vi "FRCts20_Backend_RemoveTeamEntry.vi"(8 "error in (no error)":errorcluster, 10 "Team Number":u16) -> (0 "error out":errorcluster, 2 "Status?":string)   [LabVIEW 2014, in "FRCts20_Backend_WebMethods.lvlib"]
doc: "RemoveTeam will eliminate a team from the superceding data set. All team information will be deleted."
uses:
  FRCts20_Backend_WebMethods.lvlib
  FRCts20_Backend_FGVOperation.ctl
  FRCts20_Backend_Engine.lvlib
panel:
  # "RemoveTeam will eliminate a team from the \nsuperceding data set. All team information\nwill be deleted."
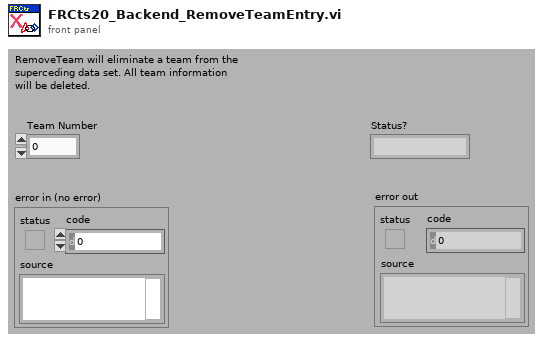
[diagram p1: front panel]
types:
  T1 = typedef "FRCts20_Backend_Engine.lvlib/FRCts20_Backend_FGVOperation.ctl" = enum16{"Initialize", "EnqueueMessage", "EnqueueDataReturn", "FlushMessage", "FlushDataReturn"}
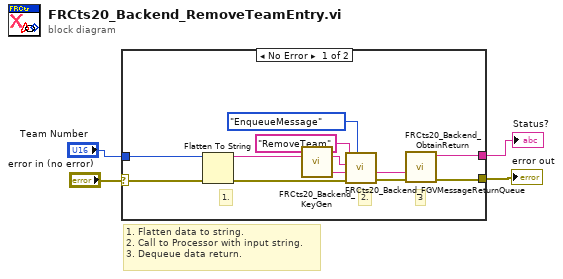
[diagram p0: block diagram]
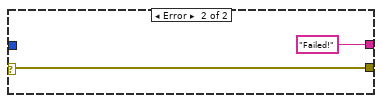
[diagram p2: hidden frame]
diagram:
  # "1. Flatten data to string.\n2. Call to Processor with input string.\n3. Dequeue data return."
  n1 = case shown="No Error" "error in (no error)" {
    selector: "error in (no error)" -> [w10 w17]
    tunnel: [w11 w17] -> w3
    tunnel: [w5 "Failed!" ("Message Value")] -> w2
    tunnel: "Team Number" -> [w8 _]
    frame No Error {
      # "3"
      # "2."
      # "1."
      n2 = Flatten To String(anything=w8, error in (no error)=w10) -> (data string=w7:string, error out=w9:errorcluster)  [unwired: 2 in, 1 out]
      n3 = call "FRCts20_Backend_KeyGen.vi"() -> ("Keygen"=w13:string)  [unwired: 27 in]
      n4 = call "FRCts20_Backend_FGVMessageReturnQueue.vi"("Operation"=FRCts20_Backend_FGVOperation."EnqueueMessage", "error in (no error)"=w9, "Key"=w13, "Message Value"=w7, "Message Name"="RemoveTeam") -> ("error out"=w12:errorcluster, "Key (Duplicate)"=w6:string)  [unwired: 3 in]
      n5 = call "FRCts20_Backend_ObtainReturn.vi"("error in (no error)"=w12, "Key"=w6) -> ("error out"=w11:errorcluster, "Message Value"=w5:string)  [unwired: 8 in]
    }
    frame Error {
    }
  }
  "error out" <- w3
  "Status?" <- w2
